vi "Example (CompactRIO).vi"() -> ()   [LabVIEW 2010]
uses:
  <vilib>/eio/EIONode/EIONode.xnode
panel:
  out "Device Temperature":i16
  in  "Stop":bool
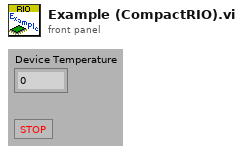
[diagram p1: front panel]
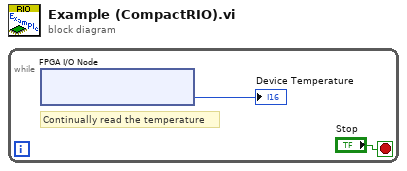
[diagram p0: block diagram]
diagram:
  n1 = while {
    stop <- "Stop" stop-if-true
    # "Continually read the temperature"
    n2 = xnode "FPGA I/O Node"() -> ("Chassis Temperature"=→"Device Temperature":i16)  [unwired: 1 in, 1 out]
  }
